vi "Read Register (U64).vi"(0 "SLSC Interface in":refnum<class "SLSC Interface.lvclass">, 5 "device":refnum<k21>="$DefaultDevices", 7 "register address":u32 format="%.0x", 11 "error in (no error)":errorcluster) -> (4 "SLSC Interface out":refnum<class "SLSC Interface.lvclass">, 6 "device out":refnum<k21>, 8 "next register address":u32 format="%.0x", 10 "data out":u64 format="%.0x", 15 "error out":errorcluster)   [LabVIEW 2016, in "SLSC Interfaces.lvlib" / "SLSC Interface.lvclass"]
uses:
  SLSC Interface.lvclass
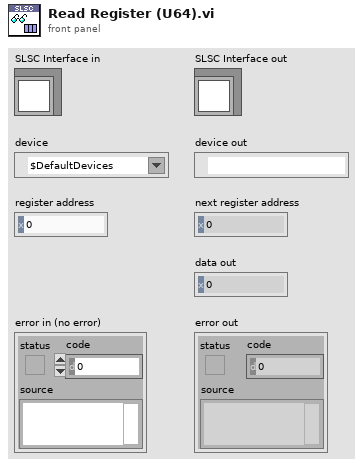
[diagram p1: front panel]
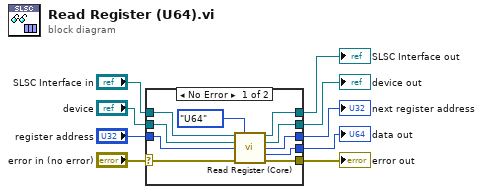
[diagram p0: block diagram]
diagram:
  n1 = case shown="No Error" "error in (no error)" {
    selector: "error in (no error)" -> [w17 w23]
    tunnel: [w16 w23] -> w8
    tunnel: [w18 w22] -> w6
    tunnel: "SLSC Interface in" -> [w19 w22]
    tunnel: "register address" -> [w11 w21]
    tunnel: [w14 w20] -> w4
    tunnel: [w13 w21] -> w3
    tunnel: [w10 _] -> w2
    tunnel: "device" -> [w12 w20]
    frame No Error {
      n2 = call "Read Register (Core).vi"("SLSC Interface in"=w19, "type"=enum16{"U8", "U16", "U32", "U64"}."U64" ("size"), "device"=w12, "register address"=w11, "error in (no error)"=w17) -> ("SLSC Interface out"=w18:refnum<class "SLSC Interface.lvclass">, "device out"=w14:refnum<k21>, "next register address"=w13:u32, "data out"=w10:u64, "error out"=w16:errorcluster)  [unwired: 6 in]
    }
    frame Error {
    }
  }
  "error out" <- w8
  "SLSC Interface out" <- w6
  "device out" <- w4
  "next register address" <- w3
  "data out" <- w2
